vi "BuildSetPacketParams.vi"(7 "UnitType":T1(ring), 8 "DevType":T2(ring), 9 "index":i32, 10 "Numeric":i32=4, 11 "Ch num":u8(ring) items=["Ch 1"]) -> (2 "Array":T3(array[cluster]))   [LabVIEW 2017]
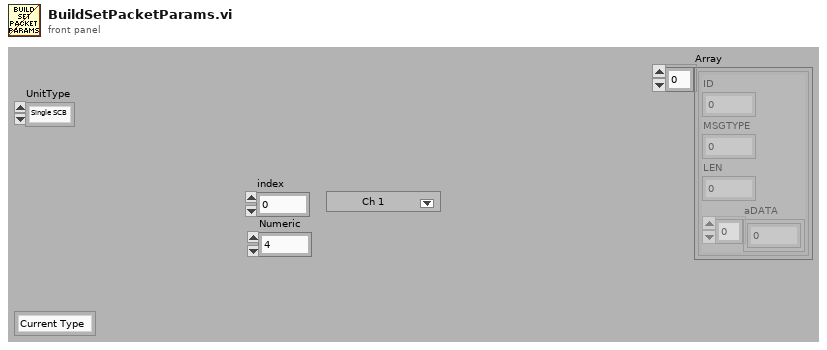
[diagram p1: front panel]
types:
  T1 = enum16{"Single SCB", "Power Rider", "Power Rider&Next10", "HATAL", "DAPH", "Indefinite", "Power Rider 12"}
  T2 = enum16{"Current Type", "Type 1", "Type 2", "Type 3", "Type 4", "Type 5", "Type 6", "Type 7", "Type 8", "Type 9", "Type 10"}
  T3 = cluster{"ID":u32, "MSGTYPE":u8, "LEN":u8, "aDATA":u8[]}[]
  T4 = cluster{"ID":u32, "MSGTYPE":u8, "LEN":u8, "aDATA":u8[]}
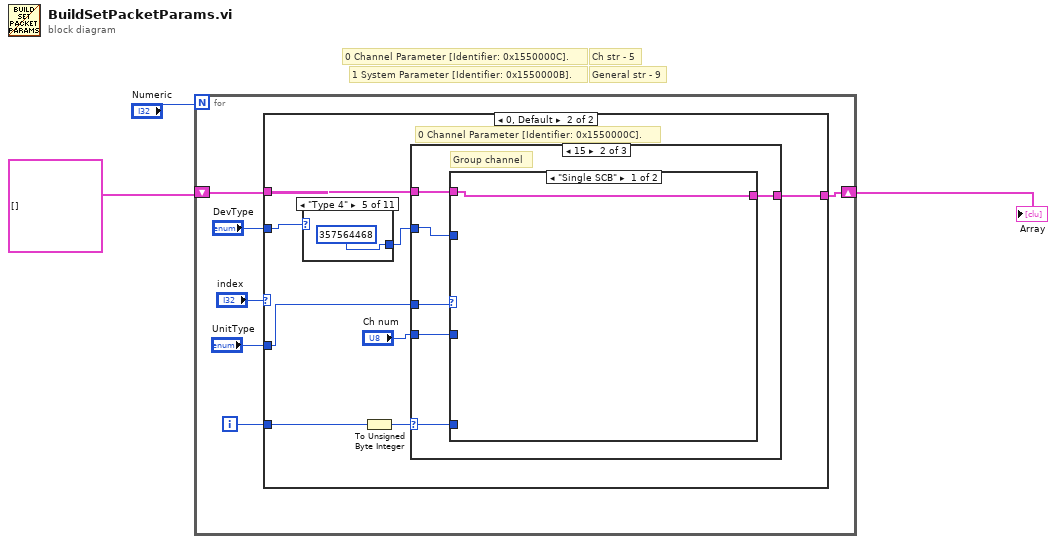
[diagram p0: block diagram]
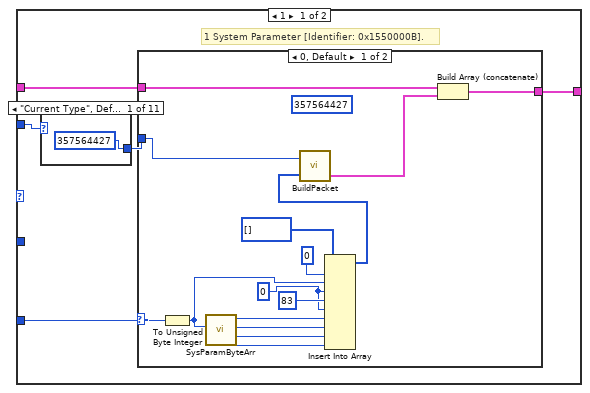
[diagram p2: hidden frame]
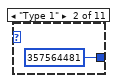
[diagram p3: hidden frame]
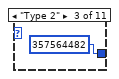
[diagram p4: hidden frame]
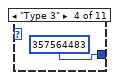
[diagram p5: hidden frame]
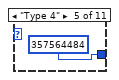
[diagram p6: hidden frame]
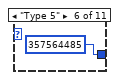
[diagram p7: hidden frame]
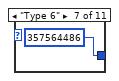
[diagram p8: hidden frame]
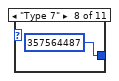
[diagram p9: hidden frame]
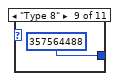
[diagram p10: hidden frame]
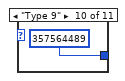
[diagram p11: hidden frame]
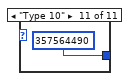
[diagram p12: hidden frame]
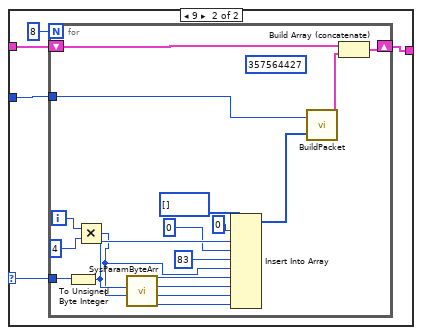
[diagram p13: hidden frame]
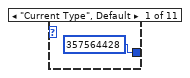
[diagram p14: hidden frame]
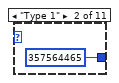
[diagram p15: hidden frame]
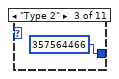
[diagram p16: hidden frame]
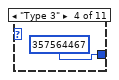
[diagram p17: hidden frame]
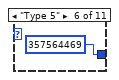
[diagram p18: hidden frame]
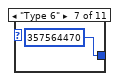
[diagram p19: hidden frame]
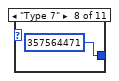
[diagram p20: hidden frame]
diagram:
  # "0 Channel Parameter [Identifier: 0x1550000C]."
  # "1 System Parameter [Identifier: 0x1550000B]."
  # "Ch str - 5"
  # "General str - 9"
  n1 = for {
    N: "Numeric" -> [_]
    shift-right: [w8] -> w1
    shift-left: T3 [] ("Array") -> [w9]
    i -> [w7]
    n2 = case shown="0, Default" "index" {
      tunnel: w9 -> [w14 w71]
      tunnel: [w13 w70] -> w8
      tunnel: w7 -> [w12 w69]
      tunnel: "DevType" -> [w11 w66]
      tunnel: "UnitType" -> [_ w64]
      frame 1 {
        # "1 System Parameter [Identifier: 0x1550000B]."
        n3 = case shown="\"Current Type\", Default" w11 {
          tunnel: [u32 357564427 u32 357564481 u32 357564482 u32 357564483 u32 357564484 u32 357564485 u32 357564486 u32 357564487 u32 357564488 u32 357564489 u32 357564490] -> w10
          frame "Current Type", Default {
          }
          frame "Type 1" {
          }
          frame "Type 2" {
          }
          frame "Type 3" {
          }
          frame "Type 4" {
          }
          frame "Type 5" {
          }
          frame "Type 6" {
          }
          frame "Type 7" {
          }
          frame "Type 8" {
          }
          frame "Type 9" {
          }
          frame "Type 10" {
          }
        }
        n4 = case shown="0, Default" w12 {
          selector: w12 -> [w35 w44]
          tunnel: w14 -> [w40 w45]
          tunnel: [w39 w43] -> w13
          tunnel: w10 -> [w26 w41]
          frame 0, Default {
            w31 = u8 0 ("index")
            (unwired) u32 357564427 ("Param ID")
            n5 = To Unsigned Byte Integer(number=w35) -> (unsigned 8bit integer=w33:u8)
            n6 = call "SysParamByteArr.vi"("Param Nm"=w33) -> ("Byte3"=w27:u8, "Byte2"=w28:u8, "Byte1"=w29:u8, "Byte0"=w30:u8)  [unwired: 7 in]
            n7 = Insert Into Array(array=u8[] [] ("Data 2"), index=0, new element #1=w33, new element #2=w31, new element #3=u8 83 ("new element/subarray"), new element #4=w31, new element #5=w30, new element #6=w29, new element #7=w28, new element #8=w27) -> (w36:u8[])
            n8 = call "BuildPacket.vi"("Data"=w36, "TxID"=w26) -> ("MsgTX 2"=w38:T4)
            n9 = Build Array (concatenate)(w40, w38) -> (w39:T3)
          }
          frame 9 {
            n10 = for {
              N: 8 -> [_]
              tunnel: w44 -> [w57]
              shift-right: [w56] -> w43
              shift-left: w45 -> [w63]
              tunnel: w41 -> [w46]
              i -> [w50]
              (unwired) u32 357564427 ("Param ID")
              n11 = To Unsigned Byte Integer(number=w57) -> (unsigned 8bit integer=w58:u8)
              n12 = Multiply(x=w50, y=4) -> (x*y=w47:i32)
              n13 = call "SysParamByteArr.vi"("idx"=w47, "Param Nm"=w58) -> ("Byte3"=w51:u8, "Byte2"=w52:u8, "Byte1"=w53:u8, "Byte0"=w54:u8)  [unwired: 6 in]
              n14 = Insert Into Array(array=u8[] [] ("Data 2"), index=0, new element #1=w58, new element #2=0 ("index"), new element #3=u8 83 ("new element/subarray"), new element #4=w47, new element #5=w54, new element #6=w53, new element #7=w52, new element #8=w51) -> (w60:u8[])
              n15 = call "BuildPacket.vi"("Data"=w60, "TxID"=w46) -> ("MsgTX 2"=w62:T4)
              n16 = Build Array (concatenate)(w63, w62) -> (w56:T3)
            }
          }
        }
      }
      frame 0, Default {
        # "0 Channel Parameter [Identifier: 0x1550000C]."
        n17 = case shown="\"Type 4\"" w66 {
          tunnel: [u32 357564428 u32 357564465 u32 357564466 u32 357564467 u32 357564468 u32 357564469 u32 357564470 u32 357564471 u32 357564472 u32 357564473 u32 357564474] -> w65
          frame "Current Type", Default {
          }
          frame "Type 1" {
          }
          frame "Type 2" {
          }
          frame "Type 3" {
          }
          frame "Type 4" {
          }
          frame "Type 5" {
          }
          frame "Type 6" {
          }
          frame "Type 7" {
          }
          frame "Type 8" {
          }
          frame "Type 9" {
          }
          frame "Type 10" {
          }
        }
        n18 = To Unsigned Byte Integer(number=w69) -> (unsigned 8bit integer=w68:u8)
        n19 = case shown="15" w68 {
          selector: w68 -> [w85 w101 w124]
          tunnel: w71 -> [w97 w103 w125]
          tunnel: [w96 w102 w122] -> w70
          tunnel: "Ch num" -> [w84 w100 w123]
          tunnel: w65 -> [w83 w99 w120]
          tunnel: w64 -> [_ w98 _]
          frame 1, Default {
            (unwired) u32 357564428 ("Param ID")
            # "\"S\"=83"
            n20 = call "ParamByteArray.vi"("Param Nm"=w85) -> ("Byte3"=w89:u8, "Byte2"=w90:u8, "Byte1"=w91:u8, "Byte0"=w92:u8)  [unwired: 4 in]
            n21 = Insert Into Array(array=u8[] [] ("Data 2"), index=0, new element #1=w85, new element #2=w84, new element #3=u8 83 ("new element/subarray"), new element #4=u8 0 ("index"), new element #5=w92, new element #6=w91, new element #7=w90, new element #8=w89) -> (w93:u8[])
            n22 = call "BuildPacket.vi"("Data"=w93, "TxID"=w83) -> ("MsgTX 2"=w95:T4)
            n23 = Build Array (concatenate)(w97, w95) -> (w96:T3)
          }
          frame 15 {
            # "Group channel"
            n24 = case shown="\"Single SCB\"" w98 {
              tunnel: w103 -> [w104 w119]
              tunnel: [w104 w118] -> w102
              tunnel: w101 -> [_ w107]
              tunnel: w100 -> [_ w106]
              tunnel: w99 -> [_ w105]
              frame "Single SCB" {
              }
              frame "Power Rider", Default {
                (unwired) u32 357564428 ("Param ID")
                # "\"S\"=83"
                n25 = call "ParamByteArray.vi"("Param Nm"=w107) -> ("Byte3"=w111:u8, "Byte2"=w112:u8, "Byte1"=w113:u8, "Byte0"=w114:u8)  [unwired: 4 in]
                n26 = Insert Into Array(array=u8[] [] ("Data 2"), index=0, new element #1=w107, new element #2=w106, new element #3=u8 83 ("new element/subarray"), new element #4=u8 0 ("index"), new element #5=w114, new element #6=w113, new element #7=w112, new element #8=w111) -> (w115:u8[])
                n27 = call "BuildPacket.vi"("Data"=w115, "TxID"=w105) -> ("MsgTX 2"=w117:T4)
                n28 = Build Array (concatenate)(w119, w117) -> (w118:T3)
              }
            }
          }
          frame 5 {
            # "Str"
            n29 = for {
              N: 8 -> [_]
              tunnel: w124 -> [w132]
              tunnel: w123 -> [w131]
              shift-right: [w130] -> w122
              shift-left: w125 -> [w142]
              tunnel: w120 -> [w126]
              i -> [w128]
              (unwired) u32 357564428 ("Param ID")
              # "\"S\"=83"
              n30 = Multiply(x=w128, y=4) -> (x*y=w127:i32)
              n31 = call "ParamByteArray.vi"("idx"=w127, "Param Nm"=w132) -> ("Byte3"=w135:u8, "Byte2"=w136:u8, "Byte1"=w137:u8, "Byte0"=w138:u8)  [unwired: 3 in]
              n32 = Insert Into Array(array=u8[] [] ("Data 2"), index=0, new element #1=w132, new element #2=w131, new element #3=u8 83 ("new element/subarray"), new element #4=w127, new element #5=w138, new element #6=w137, new element #7=w136, new element #8=w135) -> (w139:u8[])
              n33 = call "BuildPacket.vi"("Data"=w139, "TxID"=w126) -> ("MsgTX 2"=w141:T4)
              n34 = Build Array (concatenate)(w142, w141) -> (w130:T3)
            }
          }
        }
      }
    }
  }
  "Array" <- w1
